vi "Traffic Light.vi"() -> ()   [LabVIEW 2019]
uses:
  <vilib>/Platform/TimedLoop/XDataNode/timing_clust.ctl
  <vilib>/Platform/TimedLoop/XDataNode/nitl_modes.ctl
  <vilib>/Platform/TimedLoop/XDataNode/wakeup.ctl
  <vilib>/platform/TimedLoop/XDataNode/XDataNode.xnode
  <vilib>/Platform/TimedLoop/XDataNode/XDNodeRunTimeDep.lvlib
panel:
  out "Green LED":bool
  out "Yellow LED":bool
  out "Red LED":bool
  in  "Stop":bool
  # "TRAFFIC LIGHT"
  # "using JKI Framework"
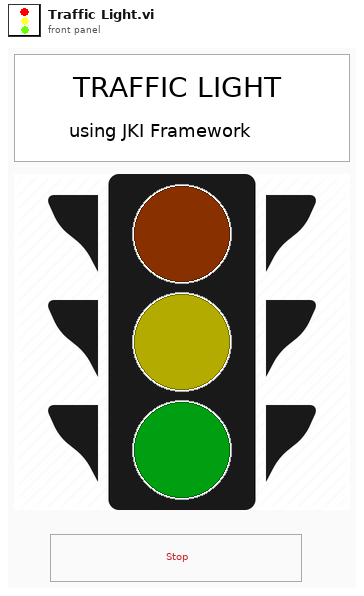
[diagram p1: front panel]
types:
  T1 = typedef "XDNodeRunTimeDep.lvlib/timing_clust.ctl" = cluster{"Expected End [f-1]":u64, "Actual End [f-1]":u64, "Finished Late? [f-1]":bool, "Expected End [i-1]":u64, "Actual End [i-1]":u64, "Finished Late? [i-1]":bool, "Expected Start [i]":u64, "Actual Start [i]":u64, "Expected Start [f]":u64, "Actual Start [f]":u64, "Source Name":string, "Structure Name":string, "Period":i64, "Deadline":i64, "Offset":i64, "Start":i64, "Priority":i32, "Timeout":i32, "Mode":T2, "Wakeup Reason":T3, "Error":errorcluster, "Source Type":string, "Secondary Source Type":string, "Global End Time":u64, "Global Start Time":u64, "Frame Duration":u64, "Iteration Duration":u64, "Assigned CPU":i32, "I/O Scan Engine Mode":u32}
  T2 = typedef "XDNodeRunTimeDep.lvlib/nitl_modes.ctl" = enum32{"No Change", "Process missed periods, maintain original phase", "Discard missed periods, maintain original phase", "Process missed periods, ignore original phase", "Discard missed periods, ignore original phase"}
  T3 = typedef "XDNodeRunTimeDep.lvlib/wakeup.ctl" = enum32{"Normal", "Aborted", "Asynchronous wakeup", "Timing source error", "Timed loop error", "Timeout"}
  T4 = enum32{"Invalid", "Standard", "Closed", "Hidden", "Minimized", "Maximized"}
  T5 = enum32{"invalid app kind", "Development System", "Run Time System", "Student Edition", "Embedded LabVIEW", "Evaluation", "Custom"}
  T6 = cluster{"Core":cluster{"Current VI Reference":refnum<vi>, "Close Panel on Exit?":bool}, "Count":i32, "Red":bool, "Yellow":bool, "Green":bool}
  T7 = cluster{"Current VI Reference":refnum<vi>, "Close Panel on Exit?":bool}
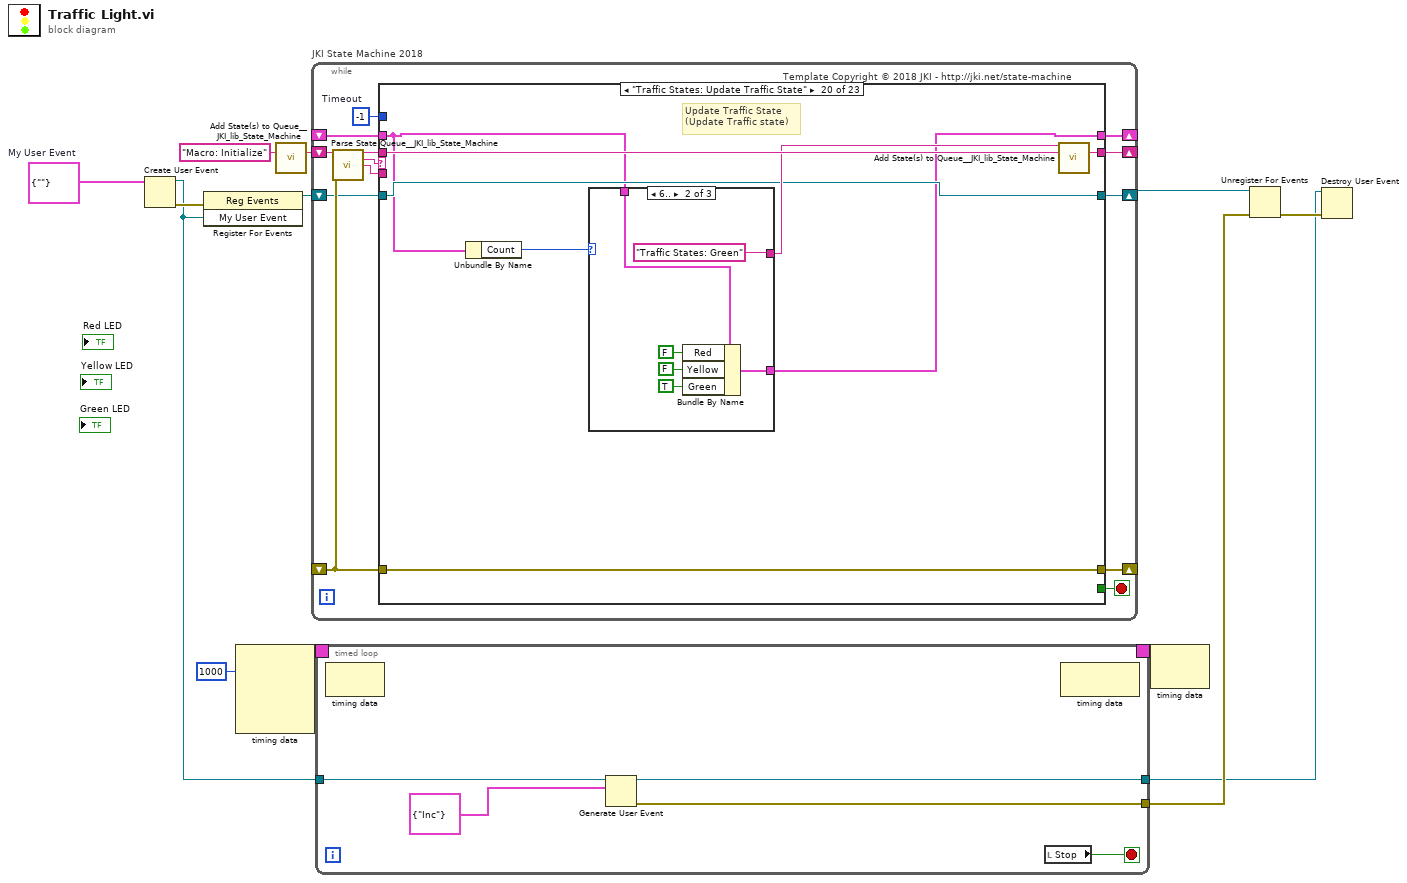
[diagram p0: block diagram]
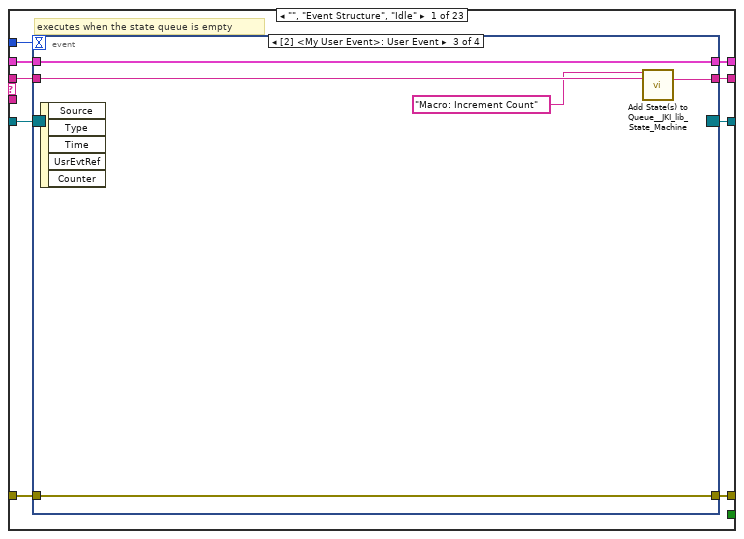
[diagram p2: hidden frame]
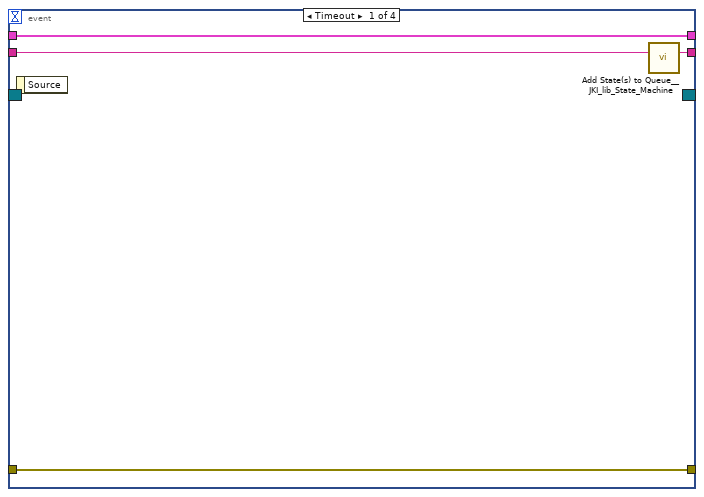
[diagram p3: hidden frame]
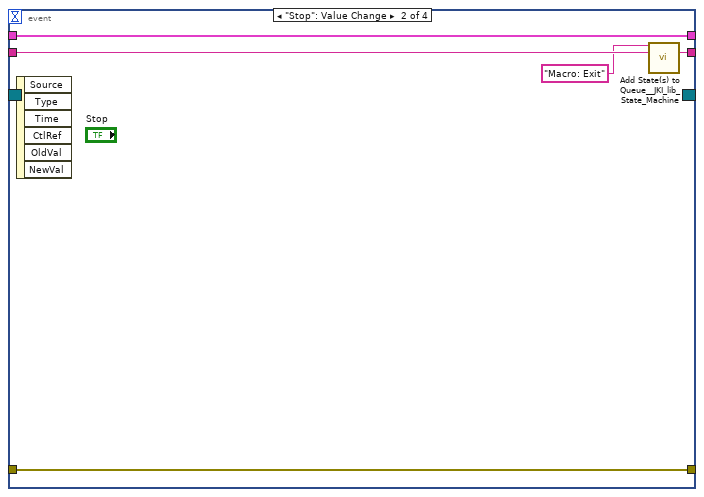
[diagram p4: hidden frame]
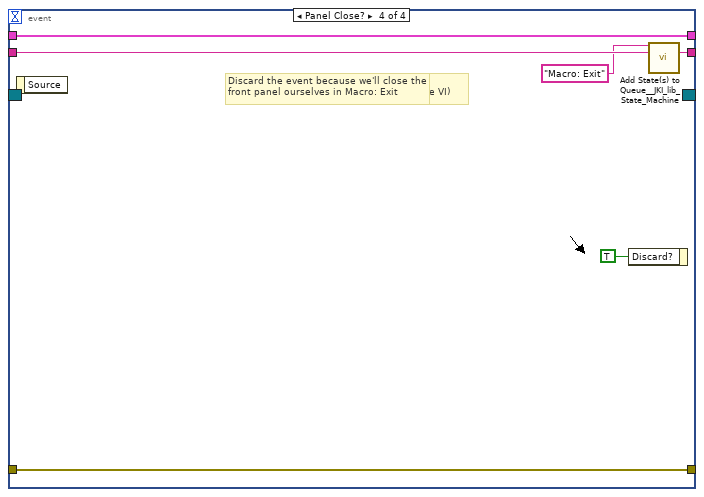
[diagram p5: hidden frame]
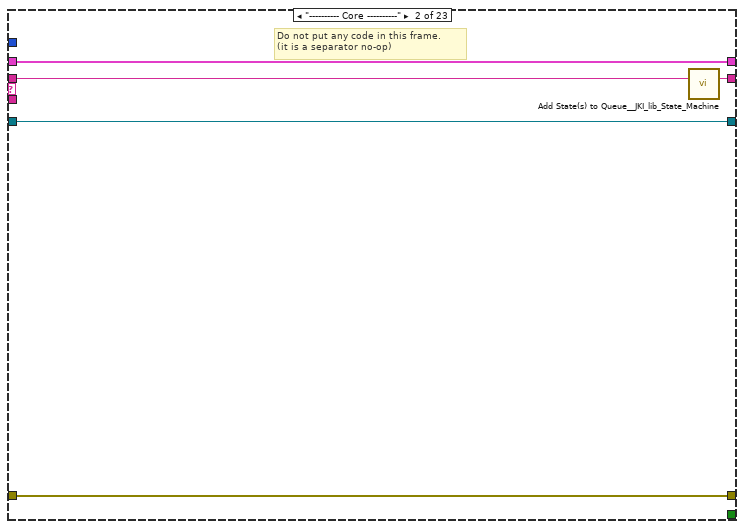
[diagram p6: hidden frame]
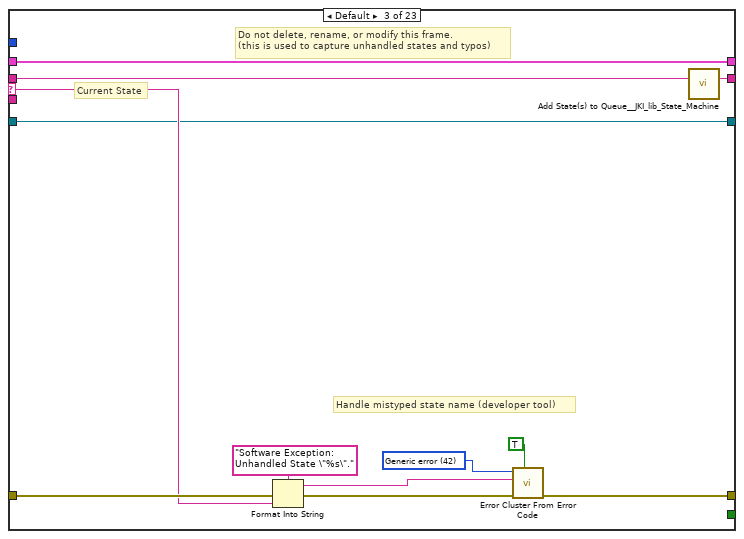
[diagram p7: hidden frame]
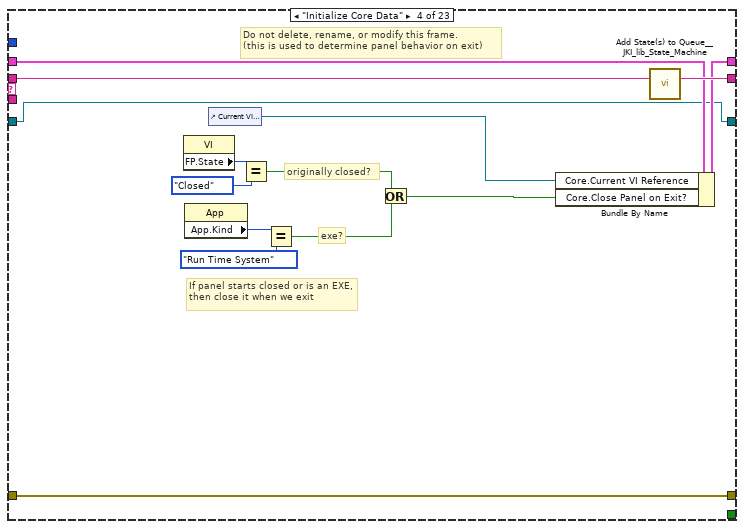
[diagram p8: hidden frame]
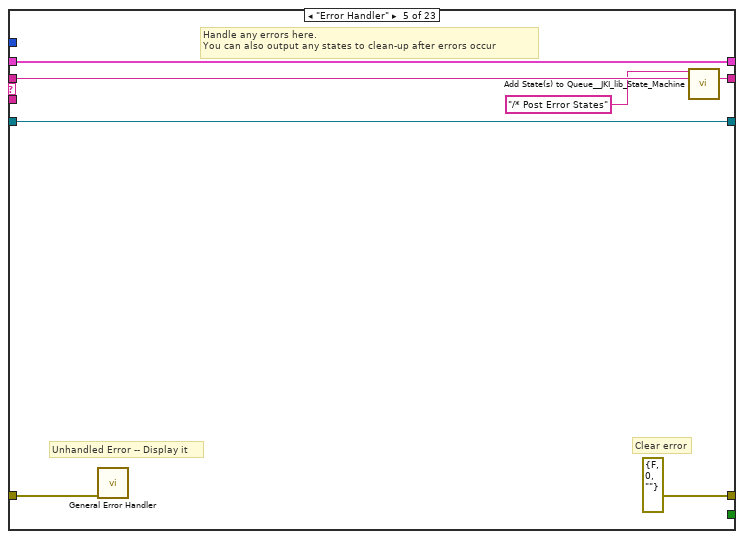
[diagram p9: hidden frame]
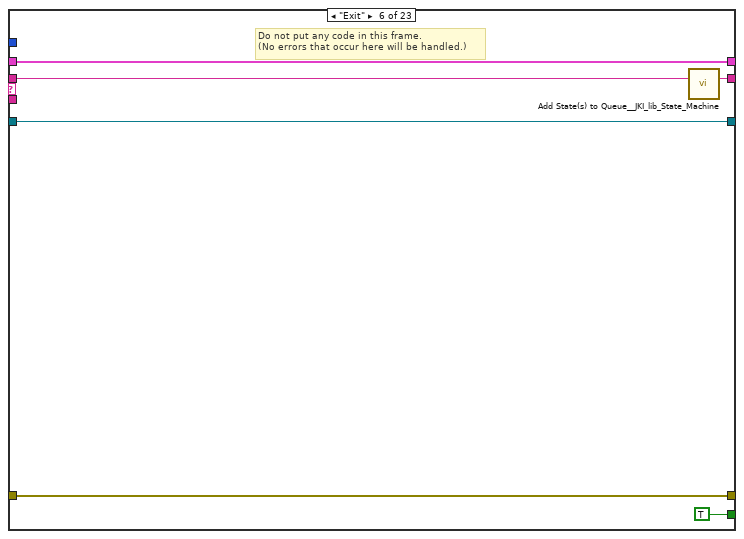
[diagram p10: hidden frame]
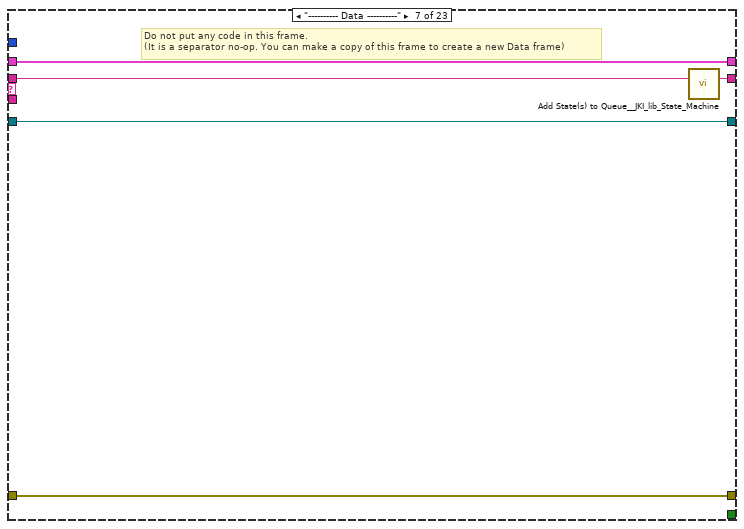
[diagram p11: hidden frame]
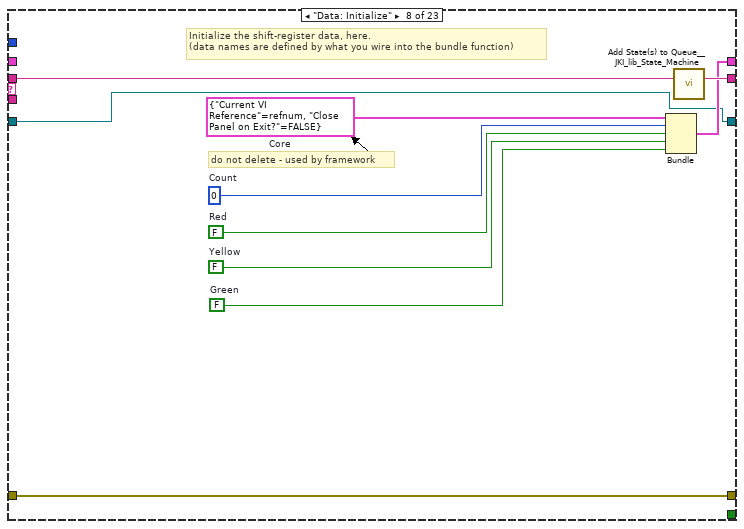
[diagram p12: hidden frame]
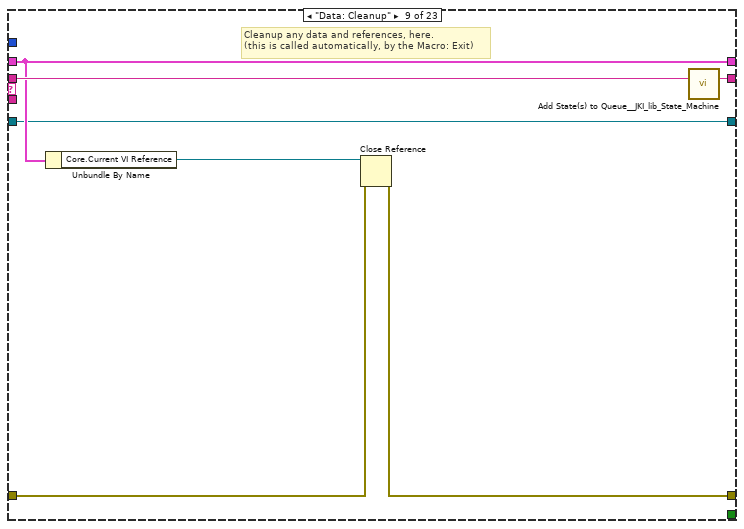
[diagram p13: hidden frame]
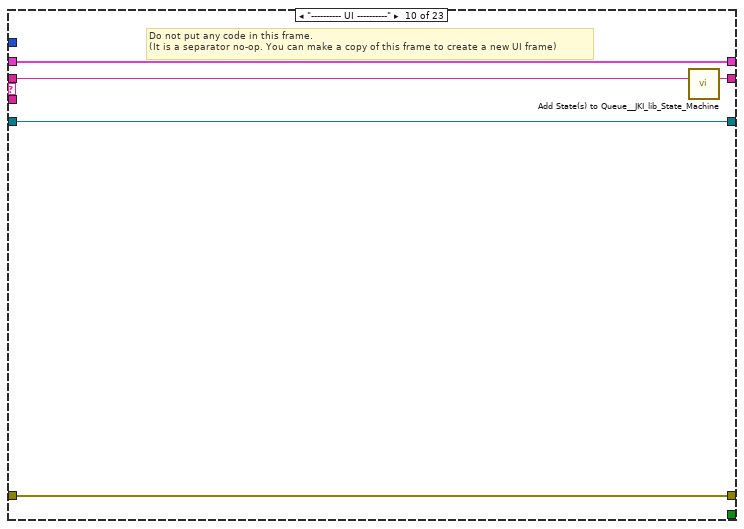
[diagram p14: hidden frame]
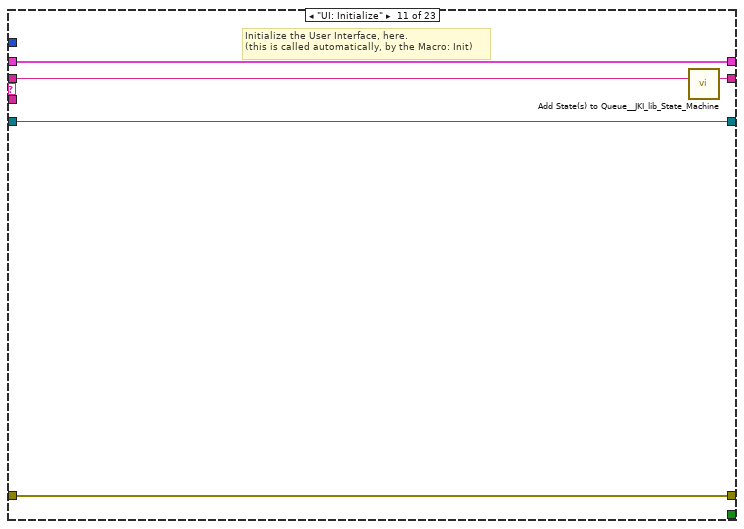
[diagram p15: hidden frame]
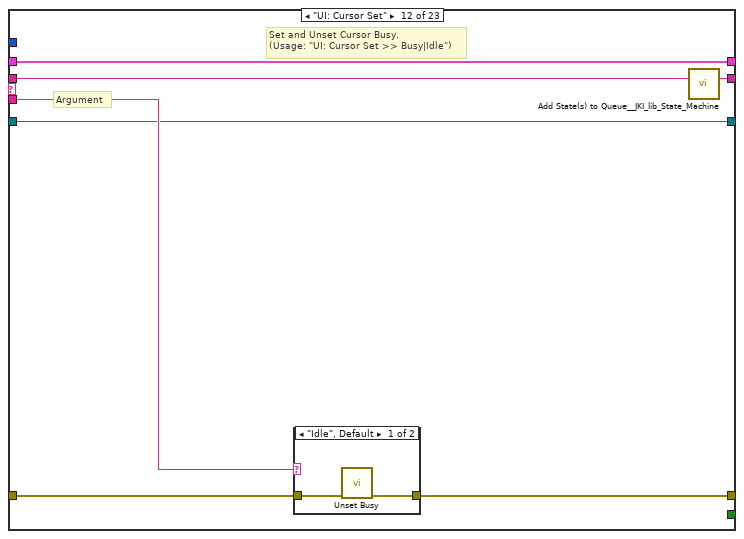
[diagram p16: hidden frame]
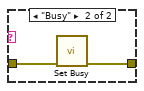
[diagram p17: hidden frame]
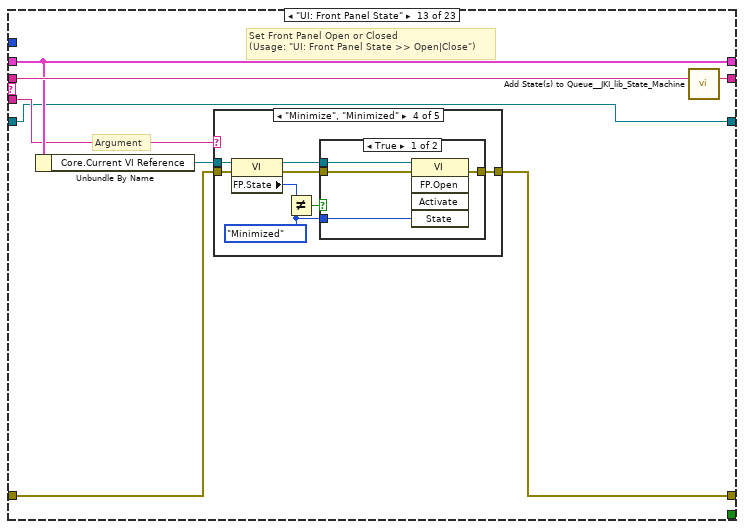
[diagram p18: hidden frame]
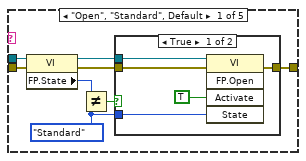
[diagram p19: hidden frame]
diagram:
  w10 = cluster{"Counter":string} {"Counter"=""}  # My User Event
  n1 = Create User Event(user event datatype=w10) -> (user event=w5:refnum<user-event>, error out=w11:errorcluster)  [unwired: 1 in]
  n2 = register-events(error in=w11, w5) -> (reference out=w9:refnum<event-registration>)  [unwired: 1 in, 1 out]
  n3 = node-c288(i64 1000 ("Period")) -> (w8:T1)  [unwired: 3 in]
  n4 = call <vilib>:"Add State(s) to Queue__JKI_lib_State_Machine.vi"("State(s) in (\"\")"="Macro: Initialize") -> ("States Out"=w13:string)  [unwired: 14 in]
  n5 = while "JKI State Machine 2018" {
    shift-right: [w19] -> _
    shift-left: _ -> [w18]
    shift-right: [w22] -> _
    shift-left: _ -> [w16]
    shift-right: [w21] -> _
    shift-left: w13 -> [w23]
    shift-right: [w14] -> w4
    shift-left: w9 -> [w15]
    stop <- w20 stop-if-true
    w17 = -1  # Timeout
    # "Template Copyright © 2018 JKI - http://jki.net/state-machine"
    n6 = call <vilib>:"Parse State Queue__JKI_lib_State_Machine.vi"("State Queue"=w23, "Error In (no error)"=w16) -> ("Remaining States"=w25:string, "Current State"=w26:string, "Arguments"=w24:string)  [unwired: 11 in]
    n7 = case shown="\"Traffic States: Update Traffic State\"" w26 {
      selector: w26 -> [_ _ w62 _ _ _ _ _ _ _ _ _ _ _ _ _ _ _ _ _ _ _ _]
      tunnel: w25 -> [w35 w60 w66 w86 w93 w99 w104 w114 w121 w126 w131 w138 w150 w220 w227 w240 w246 w258 w263 w271 w297 w305 w313]
      tunnel: w24 -> [_ _ _ _ _ _ _ _ _ _ _ w133 w144 _ _ _ _ _ _ _ _ _ _]
      tunnel: w18 -> [w33 w57 w64 w79 w90 w97 w101 _ w116 w123 w129 w136 w146 w217 w224 w232 w243 w255 w260 w264 w293 w301 w309]
      tunnel: [w32 w58 w68 w83 errorcluster {"status"=FALSE, "code"=0, "source"=""} ("error out") w96 w102 w111 w117 w124 w128 w134 w147 w218 w225 w238 w244 w256 w261 w269 w295 w303 w311] -> w22
      tunnel: w16 -> [w31 w58 w67 w83 w89 w96 w102 w111 w118 w124 w128 w135 w148 w218 w225 w238 w244 w256 w261 w269 w295 w303 w311]
      tunnel: [w34 w59 w65 w85 w92 w98 w103 w113 w120 w125 w130 w137 w149 w219 w226 w239 w245 w257 w262 w270 w296 w304 w312] -> w21
      tunnel: [_ _ _ _ _ TRUE _ _ _ _ _ _ _ _ _ _ _ TRUE _ _ _ _ _] -> w20
      tunnel: [w30 w57 w64 w84 w90 w97 w101 w112 w116 w123 w129 w136 w146 w217 w222 w231 w243 w255 w260 w265 w293 w301 w309] -> w19
      tunnel: w17 -> [w29 _ _ _ _ _ _ _ _ _ _ _ _ _ _ _ _ _ _ _ _ _ _]
      tunnel: w15 -> [w28 w56 w61 w73 w87 w94 w100 w108 w115 w122 w127 w132 w143 w216 w221 w230 w241 w247 w259 w266 w294 w302 w310]
      tunnel: [w27 w56 w61 w73 w87 w94 w100 w108 w115 w122 w127 w132 w143 w216 w221 w230 w241 w247 w259 w266 w294 w302 w310] -> w14
      frame "", "Event Structure", "Idle" {
        # "executes when the state queue is empty"
        n8 = event shown="[2] <My User Event>: User Event" {
          selector: w28 -> [_ _ _ _]
          dyn-events: [_ _ _ _] -> w27
          timeout: w29 -> [_ _ _ _]
          tunnel: w35 -> [w39 w44 w48 w55]
          tunnel: [w38 w43 w49 w54] -> w34
          tunnel: w33 -> [w36 w41 w46 w52]
          tunnel: [w37 w42 w45 w53] -> w32
          tunnel: w31 -> [w37 w42 w45 w53]
          tunnel: [w36 w41 w46 w52] -> w30
          event Timeout {
            n9 = event-data() -> ()  [unwired: 1 in, 1 out]
            n10 = call <vilib>:"Add State(s) to Queue__JKI_lib_State_Machine.vi"("State(s) in (\"\")"=w39) -> ("States Out"=w38:string)  [unwired: 14 in]
          }
          event "Stop": Value Change {
            n11 = event-data() -> ()  [unwired: 1 in, 6 out]
            n12 = call <vilib>:"Add State(s) to Queue__JKI_lib_State_Machine.vi"("State(s) in Front (\"\")"="Macro: Exit", "State(s) in (\"\")"=w44) -> ("States Out"=w43:string)  [unwired: 13 in]
          }
          event User Event {
            n13 = event-data() -> ()  [unwired: 1 in, 5 out]
            n14 = call <vilib>:"Add State(s) to Queue__JKI_lib_State_Machine.vi"("State(s) in Front (\"\")"="Macro: Increment Count" ("State(s) in Front (\"\")"), "State(s) in (\"\")"=w48) -> ("States Out"=w49:string)  [unwired: 13 in]
          }
          event Panel Close? {
            # "Discard the event because we'll close the front panel ourselves in Macro: Exit"
            # "Close Panel button (pressed) Event\n(this executes Macro: Exit to terminate the VI)"
            n15 = event-data() -> ()  [unwired: 1 in, 1 out]
            n16 = event-data("Discard?"=TRUE) -> ()  [unwired: 1 in, 1 out]
            n17 = call <vilib>:"Add State(s) to Queue__JKI_lib_State_Machine.vi"("State(s) in Front (\"\")"="Macro: Exit", "State(s) in (\"\")"=w55) -> ("States Out"=w54:string)  [unwired: 13 in]
          }
        }
      }
      frame "---------- Core ----------" {
        # "Do not put any code in this frame.\n(it is a separator no-op)"
        n18 = call <vilib>:"Add State(s) to Queue__JKI_lib_State_Machine.vi"("State(s) in (\"\")"=w60) -> ("States Out"=w59:string)  [unwired: 14 in]
      }
      frame Default {
        w71 = 42 items=["No error", "Argument error", "Memory is full", "Out of zone", "End of file", "File already open", "Generic file I/O error", "File not found", "File permission error", "Disk is full", "Duplicate path", "Too many files open", "System feature not enabled", "Resource file not found", "Cannot add resource", "Resource not found", "Image not found", "Image memory error", "Pen does not exist", "Config type invalid", "Config token not found", "Config parse error", "Config memory error", "Bad external code format", "Bad external code offset", "External code not present", "Null window", "Destroy window error", "Null menu", "Print aborted", "Bad print record", "Print driver error", "Windows error during printing", "Memory error during printing", "Print dialog error", "Generic print error", "Invalid device refnum", "Device not found", "Device parameter error", "Device unit error", "Cannot open device", "Device call aborted", "Generic error", "Cancelled by user", "Object ID too low", "Object ID too high", "Object not in heap", "Unknown heap", "Unknown object (invalid DefProc)", "Unknown object (DefProc not in table)", "Message out of range", "Invalid (null) method", "Unknown message", "Manager call not supported", "Bad address", "Network operation in progress", "Network operation timed out", "Connection is busy", "Network attribute not supported", "Network error", "Address in use", "System out of memory", "Connection aborted", "Connection refused", "Not connected", "Already connected", "Connection closed", "Initialization error (interapplication manager)", "Bad occurrence", "Wait on unbound occurrence handler", "Occurrence queue overflow", "Datalog type conflict", "Unused", "Unrecognized type (interapplication manager)", "Memory corrupt", "Failed to make temporary DLL", "Old CIN version", "Drag socket not found", "Failed to load drop-object", "Failed to register OLE object", "Failed to release OLE object", "Format specifier type mismatch", "Unknown format specifier", "Too few format specifiers", "Too many format specifiers", "Scan failed", "Newer CIN version", "Error converting to variant", "Runtime menu error", "Password tampered", "Variant attribute not found", "Incompatible variant data type", "Event data is not available", "Event Store is not present", "Occurrence is not found", "Event Queue is not created", "Event info is not available", "Refnum passed is NULL", "Error retrieving Class GUID", "Error retrieving CoClass GUID", "Error retrieving TypeLib GUID.", "Bad built application magic bytes.", "Specific driver is different from the specific driver associated with the Logical Name.", "There is no session opened to the class driver.", "Max Error", "MAX - Error with config objects", "MAX - Error loading configuration", "MAX - Group not supported"]
        # "Current State"
        # "Do not delete, rename, or modify this frame.\n(this is used to capture unhandled states and typos)"
        # "Handle mistyped state name (developer tool)"
        n19 = Format Into String(format string="Software Exception: Unhandled State \"%s\"." ("message"), error in=w67, w62) -> (resulting string=w70:string, error out=w69:errorcluster)  [unwired: 1 in]
        n20 = call <vilib>:"Error Cluster From Error Code.vi"("show call chain? (False)"=TRUE, "error in (no error)"=w69, "error message (\"\")"=w70, "error code (0)"=w71) -> ("error out"=w68:errorcluster)  [unwired: 5 in]
        n21 = call <vilib>:"Add State(s) to Queue__JKI_lib_State_Machine.vi"("State(s) in (\"\")"=w66) -> ("States Out"=w65:string)  [unwired: 14 in]
      }
      frame "Initialize Core Data" {
        # "Do not delete, rename, or modify this frame.\n(this is used to determine panel behavior on exit)"
        # "originally closed?"
        # "exe?"
        # "If panel starts closed or is an EXE, then close it when we exit"
        n22 = property class="VI"() -> ("FP.State"=w76:T4)  [unwired: 2 in, 2 out]
        n23 = property class="App"() -> ("App.Kind"=w82:T5)  [unwired: 2 in, 2 out]
        n24 = control-ref of="Current VI Reference"() -> (w77:refnum<vi>)
        n25 = Equal?(x=w76, y=T4."Closed" ("Front Panel Window:State")) -> (x = y?=w74:bool)
        n26 = Equal?(x=w82, y=T5."Run Time System" ("Application:Kind")) -> (x = y?=w80:bool)
        n27 = Or(x=w74, y=w80) -> (x .or. y?=w78:bool)
        n28 = Bundle By Name(cluster=w79, "Core.Current VI Reference"=w77, "Core.Close Panel on Exit?"=w78) -> (w84:T6)
        n29 = call <vilib>:"Add State(s) to Queue__JKI_lib_State_Machine.vi"("State(s) in (\"\")"=w86) -> ("States Out"=w85:string)  [unwired: 14 in]
      }
      frame "Error Handler" {
        # "Unhandled Error -- Display it"
        # "Handle any errors here.\nYou can also output any states to clean-up after errors occur"
        # "Clear error"
        n30 = call <vilib>:"General Error Handler.vi"("error in (no error)"=w89) -> ()  [unwired: 10 in, 5 out]
        n31 = call <vilib>:"Add State(s) to Queue__JKI_lib_State_Machine.vi"("State(s) in Front (\"\")"="/* Post Error States", "State(s) in (\"\")"=w93) -> ("States Out"=w92:string)  [unwired: 13 in]
      }
      frame "Exit" {
        # "Do not put any code in this frame.\n(No errors that occur here will be handled.)"
        n32 = call <vilib>:"Add State(s) to Queue__JKI_lib_State_Machine.vi"("State(s) in (\"\")"=w99) -> ("States Out"=w98:string)  [unwired: 14 in]
      }
      frame "---------- Data ----------" {
        # "Do not put any code in this frame.\n(It is a separator no-op. You can make a copy of this frame to create a new Data frame)"
        n33 = call <vilib>:"Add State(s) to Queue__JKI_lib_State_Machine.vi"("State(s) in (\"\")"=w104) -> ("States Out"=w103:string)  [unwired: 14 in]
      }
      frame "Data: Initialize" {
        w105 = FALSE  # Green
        w106 = FALSE  # Yellow
        w107 = FALSE  # Red
        w109 = 0  # Count
        w110 = T7 {"Current VI Reference"=refnum, "Close Panel on Exit?"=FALSE}  # Core
        # "do not delete - used by framework"
        # "Initialize the shift-register data, here.\n(data names are defined by what you wire into the bundle function)"
        n34 = Bundle("Core"=w110, "Count"=w109, "Red"=w107, "Yellow"=w106, "Green"=w105) -> (w112:T6)  [unwired: 1 in]
        n35 = call <vilib>:"Add State(s) to Queue__JKI_lib_State_Machine.vi"("State(s) in (\"\")"=w114) -> ("States Out"=w113:string)  [unwired: 14 in]
      }
      frame "Data: Cleanup" {
        # "Cleanup any data and references, here.\n(this is called automatically, by the Macro: Exit)"
        n36 = Unbundle By Name(w116) -> ("Core.Current VI Reference"=w119:refnum<vi>)
        n37 = Close Reference(reference=w119, error in (no error)=w118) -> (error out=w117:errorcluster)
        n38 = call <vilib>:"Add State(s) to Queue__JKI_lib_State_Machine.vi"("State(s) in (\"\")"=w121) -> ("States Out"=w120:string)  [unwired: 14 in]
      }
      frame "---------- UI ----------" {
        # "Do not put any code in this frame.\n(It is a separator no-op. You can make a copy of this frame to create a new UI frame)"
        n39 = call <vilib>:"Add State(s) to Queue__JKI_lib_State_Machine.vi"("State(s) in (\"\")"=w126) -> ("States Out"=w125:string)  [unwired: 14 in]
      }
      frame "UI: Initialize" {
        # "Initialize the User Interface, here.\n(this is called automatically, by the Macro: Init)"
        n40 = call <vilib>:"Add State(s) to Queue__JKI_lib_State_Machine.vi"("State(s) in (\"\")"=w131) -> ("States Out"=w130:string)  [unwired: 14 in]
      }
      frame "UI: Cursor Set" {
        # "Argument"
        # "Set and Unset Cursor Busy.\n(Usage: \"UI: Cursor Set >> Busy|Idle\")"
        n41 = case shown="\"Idle\", Default" w133 {
          tunnel: w135 -> [w140 w142]
          tunnel: [w139 w141] -> w134
          frame "Idle", Default {
            n42 = call <vilib>:"Unset Busy.vi"("error in (no error)"=w140) -> ("error out"=w139:errorcluster)  [unwired: 10 in]
          }
          frame "Busy" {
            n43 = call <vilib>:"Set Busy.vi"("error in (no error)"=w142) -> ("error out"=w141:errorcluster)  [unwired: 9 in, 1 out]
          }
        }
        n44 = call <vilib>:"Add State(s) to Queue__JKI_lib_State_Machine.vi"("State(s) in (\"\")"=w138) -> ("States Out"=w137:string)  [unwired: 14 in]
      }
      frame "UI: Front Panel State" {
        # "Argument"
        # "Set Front Panel Open or Closed\n(Usage: \"UI: Front Panel State >> Open|Close\")"
        n45 = Unbundle By Name(w146) -> ("Core.Current VI Reference"=w145:refnum<vi>)
        n46 = case shown="\"Minimize\", \"Minimized\"" w144 {
          tunnel: w148 -> [w156 w171 w182 w195 w208]
          tunnel: [w158 w172 w184 w197 w210] -> w147
          tunnel: w145 -> [w157 w169 w183 w196 w209]
          frame "Open", "Standard", Default {
            w151 = T4."Standard" ("State")
            n47 = property class="VI"(reference=w157, error in=w156) -> (reference out=w154:refnum<vi>, error out=w155:errorcluster, "FP.State"=w153:T4)
            n48 = Not Equal?(x=w153, y=w151) -> (x != y?=w152:bool)
            n49 = case shown="True" w152 {
              tunnel: [w162 w164] -> w158
              tunnel: w155 -> [w161 w164]
              tunnel: w154 -> [w160 _]
              tunnel: w151 -> [w159 _]
              frame True {
                n50 = invoke class="VI" method="FP.Open"(reference=w160, error in=w161, "Activate"=TRUE, "State"=w159) -> (error out=w162:errorcluster)  [unwired: 1 in, 4 out]
              }
              frame False {
              }
            }
          }
          frame "Close", "Closed" {
            n51 = property class="VI"(reference=w169, error in=w171) -> (reference out=w168:refnum<vi>, error out=w170:errorcluster, "FP.State"=w166:T4)
            n52 = Not Equal?(x=w166, y=T4."Closed" ("Front Panel Window:State")) -> (x != y?=w165:bool)
            n53 = case shown="True" w165 {
              tunnel: [w173 w176] -> w172
              tunnel: w170 -> [w173 w175]
              tunnel: w168 -> [_ w174]
              frame False {
              }
              frame True {
                n54 = invoke class="VI" method="FP.Close"(reference=w174, error in=w175) -> (error out=w176:errorcluster)  [unwired: 1 in, 2 out]
              }
            }
          }
          frame "Hidden", "Hide" {
            w177 = T4."Hidden" ("State")
            n55 = property class="VI"(reference=w183, error in=w182) -> (reference out=w180:refnum<vi>, error out=w181:errorcluster, "FP.State"=w179:T4)
            n56 = Not Equal?(x=w179, y=w177) -> (x != y?=w178:bool)
            n57 = case shown="True" w178 {
              tunnel: [w188 w189] -> w184
              tunnel: w181 -> [w187 w189]
              tunnel: w180 -> [w186 _]
              tunnel: w177 -> [w185 _]
              frame True {
                n58 = invoke class="VI" method="FP.Open"(reference=w186, error in=w187, "State"=w185) -> (error out=w188:errorcluster)  [unwired: 2 in, 4 out]
              }
              frame False {
              }
            }
          }
          frame "Minimize", "Minimized" {
            w190 = T4."Minimized" ("State")
            n59 = property class="VI"(reference=w196, error in=w195) -> (reference out=w193:refnum<vi>, error out=w194:errorcluster, "FP.State"=w192:T4)
            n60 = Not Equal?(x=w192, y=w190) -> (x != y?=w191:bool)
            n61 = case shown="True" w191 {
              tunnel: [w201 w202] -> w197
              tunnel: w194 -> [w200 w202]
              tunnel: w193 -> [w199 _]
              tunnel: w190 -> [w198 _]
              frame True {
                n62 = invoke class="VI" method="FP.Open"(reference=w199, error in=w200, "State"=w198) -> (error out=w201:errorcluster)  [unwired: 2 in, 4 out]
              }
              frame False {
              }
            }
          }
          frame "Maximize", "Maximized" {
            w203 = T4."Maximized" ("State")
            n63 = property class="VI"(reference=w209, error in=w208) -> (reference out=w206:refnum<vi>, error out=w207:errorcluster, "FP.State"=w205:T4)
            n64 = Not Equal?(x=w205, y=w203) -> (x != y?=w204:bool)
            n65 = case shown="True" w204 {
              tunnel: [w214 w215] -> w210
              tunnel: w207 -> [w213 w215]
              tunnel: w206 -> [w212 _]
              tunnel: w203 -> [w211 _]
              frame True {
                n66 = invoke class="VI" method="FP.Open"(reference=w212, error in=w213, "State"=w211) -> (error out=w214:errorcluster)  [unwired: 2 in, 4 out]
              }
              frame False {
              }
            }
          }
        }
        n67 = call <vilib>:"Add State(s) to Queue__JKI_lib_State_Machine.vi"("State(s) in (\"\")"=w150) -> ("States Out"=w149:string)  [unwired: 14 in]
      }
      frame "---------- Macro ----------" {
        # "Do not put any code in this frame.\n(It is a separator no-op. You can make a copy of this frame to create a new Macro frame)"
        n68 = call <vilib>:"Add State(s) to Queue__JKI_lib_State_Machine.vi"("State(s) in (\"\")"=w220) -> ("States Out"=w219:string)  [unwired: 14 in]
      }
      frame "Macro: Reset Count" {
        # "Reset Count\n(Reset count to 0)"
        n69 = Bundle By Name(cluster=w224, "Count"=0) -> (w222:T6)
        n70 = call <vilib>:"Add State(s) to Queue__JKI_lib_State_Machine.vi"("State(s) in (\"\")"=w227) -> ("States Out"=w226:string)  [unwired: 14 in]
      }
      frame "Macro: Increment Count" {
        # "Reset counter if > 10"
        # "Increment Count\n(Increment count every 1 second and check current count)"
        n71 = Unbundle By Name(w232) -> ("Count"=w234:i32)
        n72 = Increment(x=w234) -> (x+1=w228:i32)
        n73 = Greater?(x=w228, y=10) -> (0:w237:bool)
        n74 = Select(t=0, s=w237, f=w228) -> (s? t:f=w233:i32)
        n75 = Bundle By Name(cluster=w232, "Count"=w233) -> (w231:T6)
        n76 = call <vilib>:"Add State(s) to Queue__JKI_lib_State_Machine.vi"("State(s) in Front (\"\")"="Traffic States: Update Traffic State" ("State(s) in Front (\"\")"), "State(s) in (\"\")"=w240) -> ("States Out"=w239:string)  [unwired: 13 in]
      }
      frame "Macro: Initialize" {
        # "Initialization Macro\n(This is called once, when the VI starts)"
        n77 = call <vilib>:"Add State(s) to Queue__JKI_lib_State_Machine.vi"("State(s) in Front (\"\")"="Data: Initialize\nInitialize Core Data\nUI: Initialize\nUI: Front Panel State >> Open", "State(s) in (\"\")"=w246) -> ("States Out"=w245:string)  [unwired: 13 in]
      }
      frame "Macro: Exit" {
        # "Exit Macro\n(This is called once, when the VI exits)"
        n78 = Unbundle By Name(w255) -> ("Core.Close Panel on Exit?"=w254:bool)
        n79 = Select(t="UI: Front Panel State >> Close", s=w254, f="") -> (s? t:f=w251:string)
        n80 = call <vilib>:"Add State(s) to Queue__JKI_lib_State_Machine.vi"("State(s) in (\"\")"=w251, "State(s) at Back (\"\")"="Data: Cleanup\nExit") -> ("States Out"=w249:string)  [unwired: 13 in]
        n81 = call <vilib>:"Add State(s) to Queue__JKI_lib_State_Machine.vi"("State(s) in Front (\"\")"=w249, "State(s) in (\"\")"=w258) -> ("States Out"=w257:string)  [unwired: 13 in]
      }
      frame "---------- Traffic States ----------" {
        # "Template Separator\n(You can make a copy of, or modify, this frame)"
        n82 = call <vilib>:"Add State(s) to Queue__JKI_lib_State_Machine.vi"("State(s) in (\"\")"=w263) -> ("States Out"=w262:string)  [unwired: 14 in]
      }
      frame "Traffic States: Update Traffic State" {
        # "Update Traffic State\n(Update Traffic state)"
        n83 = Unbundle By Name(w264) -> ("Count"=w268:i32)
        n84 = case shown="6.." w268 {
          tunnel: ["Traffic States: Yellow" "Traffic States: Green" "Traffic States: Red"] -> w267
          tunnel: w264 -> [w272 w282 w284]
          tunnel: [w273 w278 w285] -> w265
          frame 4, 5 {
            n85 = Bundle By Name(cluster=w272, "Red"=FALSE, "Yellow"=TRUE, "Green"=FALSE) -> (w273:T6)
          }
          frame 6.. {
            n86 = Bundle By Name(cluster=w282, "Red"=FALSE, "Yellow"=FALSE, "Green"=TRUE) -> (w278:T6)
          }
          frame ..3, Default {
            n87 = Bundle By Name(cluster=w284, "Red"=TRUE, "Yellow"=FALSE, "Green"=FALSE) -> (w285:T6)
          }
        }
        n88 = call <vilib>:"Add State(s) to Queue__JKI_lib_State_Machine.vi"("State(s) in Front (\"\")"=w267, "State(s) in (\"\")"=w271) -> ("States Out"=w270:string)  [unwired: 13 in]
      }
      frame "Traffic States: Green" {
        # "Template Separator\n(You can make a copy of, or modify, this frame)"
        n89 = Unbundle By Name(w293) -> ("Red"=w292:bool, "Yellow"=w291:bool, "Green"=w290:bool)
        n90 = local write "Red LED"(w292) -> ()
        n91 = local write "Yellow LED"(w291) -> ()
        n92 = local write "Green LED"(w290) -> ()
        n93 = call <vilib>:"Add State(s) to Queue__JKI_lib_State_Machine.vi"("State(s) in (\"\")"=w297) -> ("States Out"=w296:string)  [unwired: 14 in]
      }
      frame "Traffic States: Red" {
        # "Your code here.\n(You can make a copy of, or modify, this frame)"
        n94 = Unbundle By Name(w301) -> ("Red"=w300:bool, "Yellow"=w299:bool, "Green"=w298:bool)
        n95 = local write "Red LED"(w300) -> ()
        n96 = local write "Yellow LED"(w299) -> ()
        n97 = local write "Green LED"(w298) -> ()
        n98 = call <vilib>:"Add State(s) to Queue__JKI_lib_State_Machine.vi"("State(s) in (\"\")"=w305) -> ("States Out"=w304:string)  [unwired: 14 in]
      }
      frame "Traffic States: Yellow" {
        # "Your code here.\n(You can make a copy of, or modify, this frame)"
        n99 = Unbundle By Name(w309) -> ("Red"=w308:bool, "Yellow"=w307:bool, "Green"=w306:bool)
        n100 = local write "Red LED"(w308) -> ()
        n101 = local write "Yellow LED"(w307) -> ()
        n102 = local write "Green LED"(w306) -> ()
        n103 = call <vilib>:"Add State(s) to Queue__JKI_lib_State_Machine.vi"("State(s) in (\"\")"=w313) -> ("States Out"=w312:string)  [unwired: 14 in]
      }
    }
  }
  n104 = timed-loop {
    timing: w8 -> [_]
    timing-out: [_] -> w7
    tunnel: w5 -> [w317]
    tunnel: [w315] -> w1
    tunnel: [w314] -> w3
    stop <- w318 stop-if-true
    n105 = node-c288() -> ()  [unwired: 1 in, 1 out]
    n106 = Generate User Event(user event=w317, event data cluster=cluster{"Counter":string} {"Counter"="Inc"} ("event data")) -> (user event out=w315:refnum<user-event>, error out=w314:errorcluster)  [unwired: 2 in]
    n107 = local read "Stop"() -> (w318:bool)
    n108 = node-c288() -> ()  [unwired: 1 in, 1 out]
  }
  n109 = node-c288(w7) -> ()  [unwired: 1 out]
  n110 = Unregister For Events(event registration refnum=w4, error in=w3) -> (error out=w2:errorcluster)
  n111 = Destroy User Event(user event=w1, error in=w2) -> ()  [unwired: 1 out]
